vi "Reset IED Status DVR.vi"(8 "error in":errorcluster, 11 "SCADA in":refnum<class "EMS Generic.lvclass">) -> (0 "error out":errorcluster, 3 "dup SCADA out":refnum<class "EMS Generic.lvclass">)   [LabVIEW 2018, in "EMS Generic Actor.lvlib" / "EMS Generic.lvclass"]
doc: "Empties the contents of the IED Status DVR"
uses:
  EMS Generic.lvclass
  EMS Generic.lvclass/EMS Generic.ctl
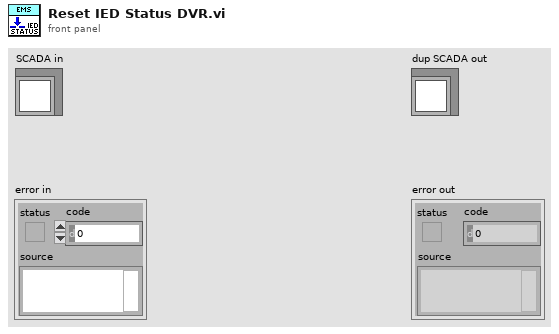
[diagram p1: front panel]
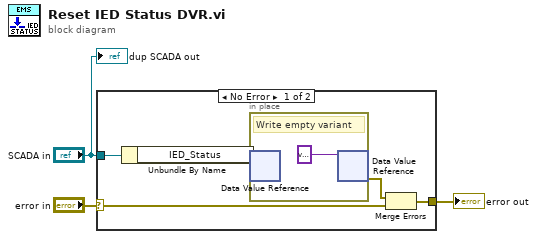
[diagram p0: block diagram]
diagram:
  n1 = case shown="No Error" "error in" {
    selector: "error in" -> [w5 w10]
    tunnel: [w4 w10] -> w2
    tunnel: "SCADA in" -> [w8 _]
    frame No Error {
      n2 = Unbundle By Name(w8) -> ("IED_Status"=w7:refnum<data-value>)
      n3 = in-place {
        # "Write empty variant"
        n4 = in-place-dvr #1(w7) -> ()  [unwired: 2 out]
        n5 = in-place-dvr #1(variant ("data value")) -> (w6:errorcluster)  [unwired: 1 out]
      }
      n6 = Merge Errors(w6, w5) -> (w4:errorcluster)
    }
    frame Error {
    }
  }
  "error out" <- w2
  "dup SCADA out" <- "SCADA in"
